vi "HEX to Normal string.vi"(1 "input hex string":string="0100") -> (0 "String":string)   [LabVIEW 2023]
panel:
  out "output normal string":string
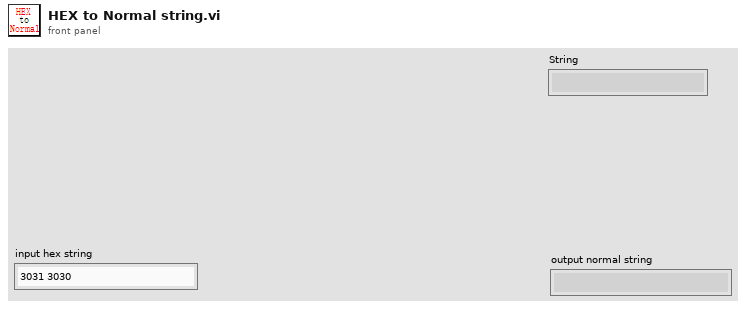
[diagram p1: front panel]
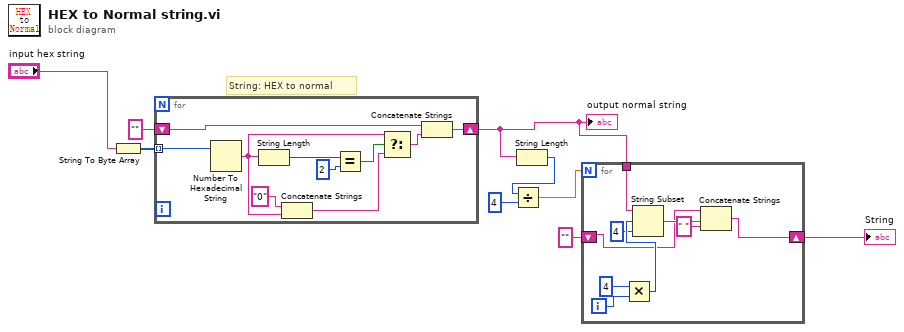
[diagram p0: block diagram]
diagram:
  # "String: HEX to normal"
  n1 = String To Byte Array(string="input hex string") -> (unsigned byte array=w9:u8[])
  n2 = for {
    tunnel: w9 -> [w19] mode=indexing
    shift-right: [w10] -> w3
    shift-left: "" -> [w12]
    n3 = Number To Hexadecimal String(2:w19) -> (0:w15:string)  [unwired: 1 in]
    n4 = String Length(string=w15) -> (length=w18:i32)
    n5 = Concatenate Strings("0" ("string"), w15) -> (w13:string)
    n6 = Equal?(x=w18, y=2) -> (x = y?=w16:bool)
    n7 = Select(t=w15, s=w16, f=w13) -> (s? t:f=w11:string)
    n8 = Concatenate Strings(w12, w11) -> (w10:string)
  }
  "output normal string" <- w3
  n9 = String Length(string=w3) -> (length=w6:i32)
  n10 = Divide(x=w6, y=4) -> (x/y=w4:dbl)
  n11 = for {
    N: w4 -> [_]
    tunnel: w3 -> [w24]
    shift-right: [w21] -> w1
    shift-left: "" -> [w20]
    i -> [w28]
    n12 = Multiply(x=4, y=w28) -> (x*y=w26:i32)
    n13 = String Subset(string=w24, offset (0)=w26, length (rest)=4 ("length (rest)")) -> (substring=w23:string)
    n14 = Concatenate Strings(w20, w23, " " ("string")) -> (w21:string)
  }
  "String" <- w1
